vi "Set Enable.vi"(7 "Enable?":bool, 11 "UI Controls":refnum<vi>[](array[refnum])) -> ()   [LabVIEW 2016]
doc: "Enable or Disable controls. Wire True means Enable while False means Disable"
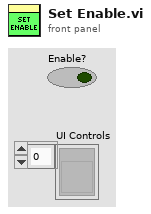
[diagram p1: front panel]
types:
  T1 = enum8{"Enabled", "Disabled", "Disabled and Grayed Out"}
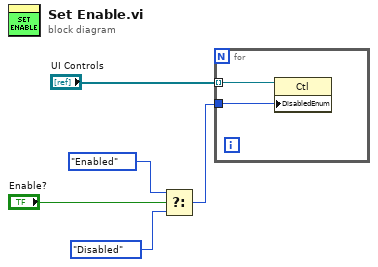
[diagram p0: block diagram]
diagram:
  n1 = Select(t=T1."Enabled" ("Enabled State"), s="Enable?", f=T1."Disabled" ("Enabled State")) -> (s? t:f=w1:T1)
  n2 = for {
    tunnel: "UI Controls" -> [w7] mode=indexing
    tunnel: w1 -> [w6]
    n3 = property class="Ctl"(reference=w7, "DisabledEnum"=w6) -> ()  [unwired: 1 in, 2 out]
  }
